vi "Time Logic.vi"(11 "Shift":string="B") -> (2 "TO":string, 3 "From":string)   [LabVIEW 2017]
panel:
  out "date/time string":string
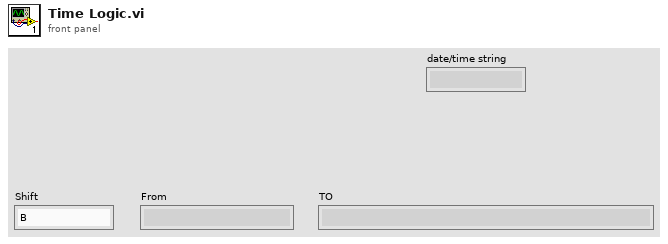
[diagram p1: front panel]
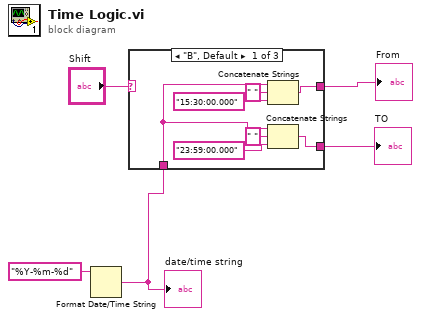
[diagram p0: block diagram]
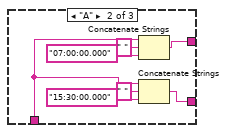
[diagram p2: hidden frame]
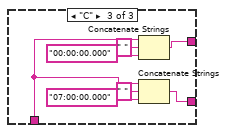
[diagram p3: hidden frame]
diagram:
  n1 = Format Date/Time String(time format string (%c)="%Y-%m-%d") -> (date/time string=w1:string)  [unwired: 2 in]
  "date/time string" <- w1
  n2 = case shown="\"B\", Default" "Shift" {
    tunnel: [w12 w19 w26] -> w5
    tunnel: w1 -> [w7 w14 w21]
    tunnel: [w8 w13 w20] -> w3
    frame "B", Default {
      n3 = Concatenate Strings(w7, " " ("string"), "15:30:00.000" ("string")) -> (w12:string)
      n4 = Concatenate Strings(w7, " " ("string"), "23:59:00.000" ("string")) -> (w8:string)
    }
    frame "A" {
      n5 = Concatenate Strings(w14, " " ("string"), "07:00:00.000" ("string")) -> (w19:string)
      n6 = Concatenate Strings(w14, " " ("string"), "15:30:00.000" ("string")) -> (w13:string)
    }
    frame "C" {
      n7 = Concatenate Strings(w21, " " ("string"), "00:00:00.000" ("string")) -> (w26:string)
      n8 = Concatenate Strings(w21, " " ("string"), "07:00:00.000" ("string")) -> (w20:string)
    }
  }
  "From" <- w5
  "TO" <- w3
